vi "page1.vi"() -> ()   [LabVIEW 2013]
uses:
  App Buttons.ctl
panel:
  in  "OK Button 11":T1
  in  "OK Button 10":T1
  in  "OK Button 9":T1
  in  "OK Button 8":T1
  in  "OK Button 7":T1
  in  "OK Button 6":T1
  in  "OK Button 5":T1
  in  "OK Button 4":T1
  in  "OK Button 3":T1
  in  "OK Button 2":T1
  in  "stop":bool
  out "Boolean":bool
  # "Page 1"
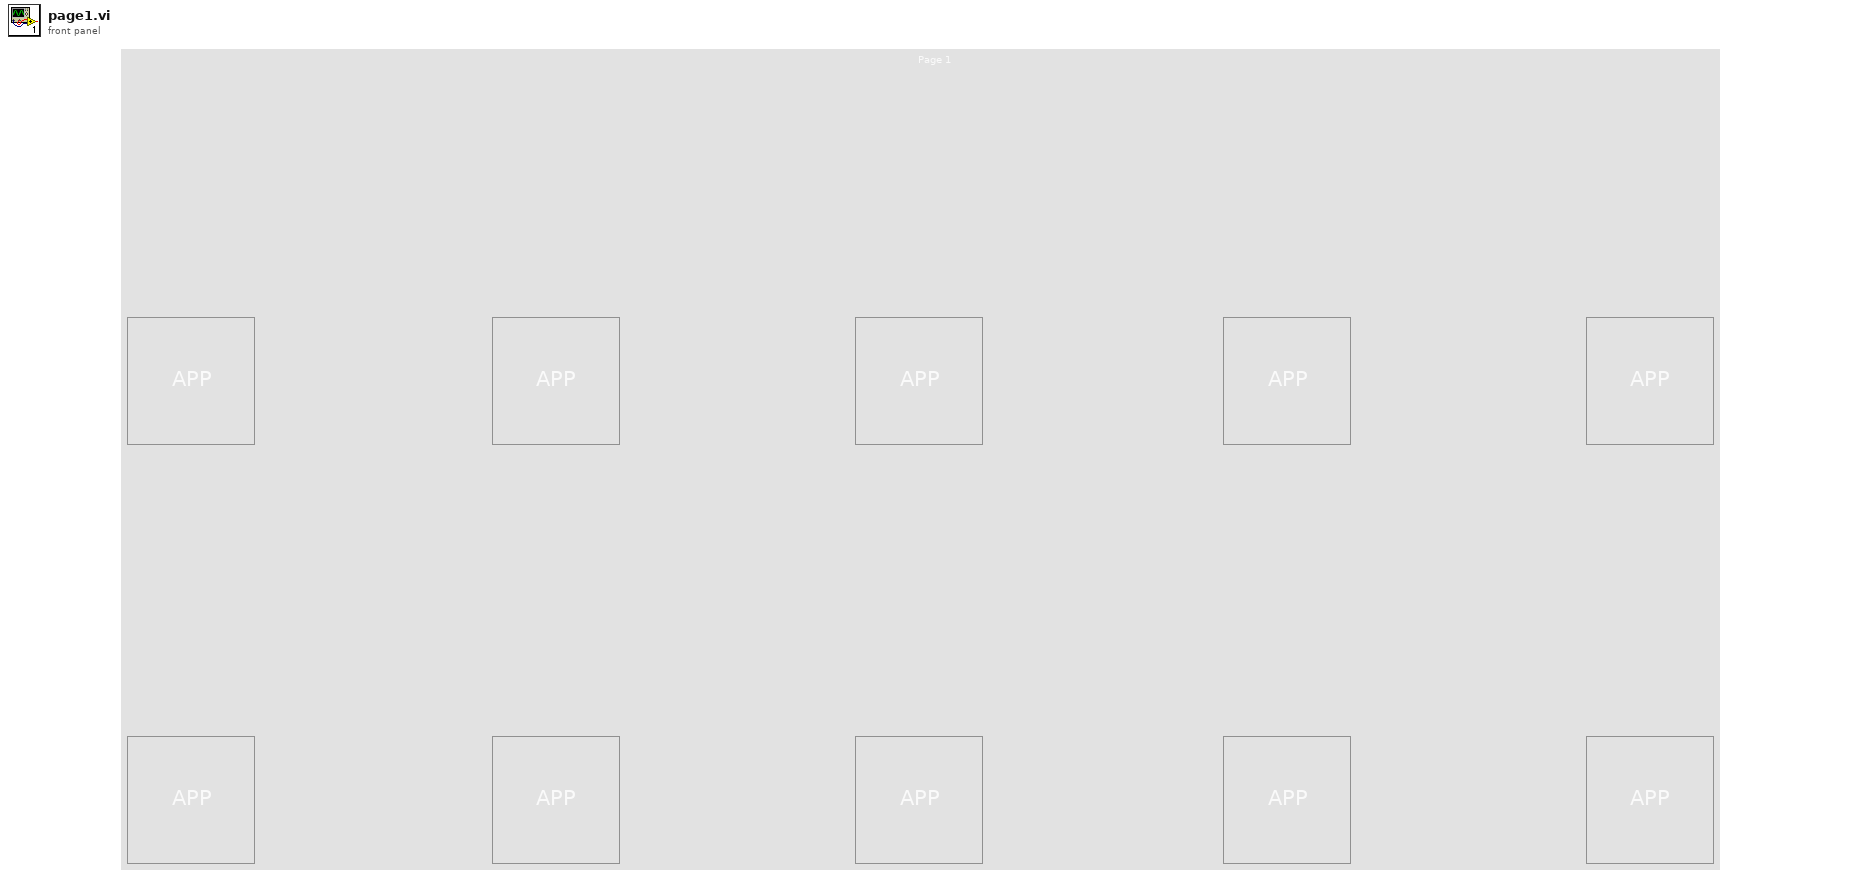
[diagram p1: front panel]
types:
  T1 = typedef "App Buttons.ctl" = bool
  T2 = typedef "imagedata.ctl" = cluster{"image type":i32, "image depth":i32, "image":u8[], "mask":u8[], "colors":u32[], "Rectangle":cluster{"left":i16, "top":i16, "right":i16, "bottom":i16}}
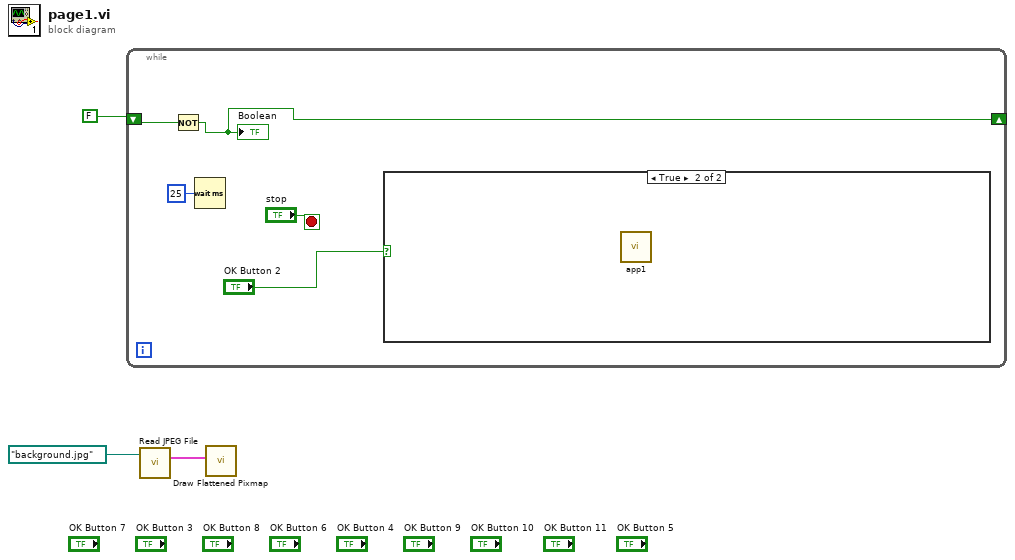
[diagram p0: block diagram]
diagram:
  n1 = while {
    shift-right: [w6] -> _
    shift-left: FALSE ("Boolean") -> [w7]
    stop <- "stop" stop-if-true
    n2 = Not(x=w7) -> (.not. x?=w6:bool)
    "Boolean" <- w6
    n3 = Wait (ms)(milliseconds to wait=u32 25) -> ()  [unwired: 1 out]
    n4 = case shown="True" "OK Button 2" {
      frame False {
      }
      frame True {
        n5 = call "app1.vi"() -> ()  [unwired: 12 in]
      }
    }
  }
  n6 = call <vilib>:"Read JPEG File.vi"("path to JPEG file"=path "background.jpg") -> ("image data"=w1:T2)  [unwired: 8 in, 2 out]
  n7 = call <vilib>:"Draw Flattened Pixmap.vi"("image data"=w1) -> ()  [unwired: 8 in, 1 out]
